vi "Untitled 1 (SubVI).vi"(0 "Message Maker in":refnum<class "Message Maker.lvclass">) -> (19 "error out":errorcluster)   [LabVIEW 2023]
uses:
  Message Maker.lvclass
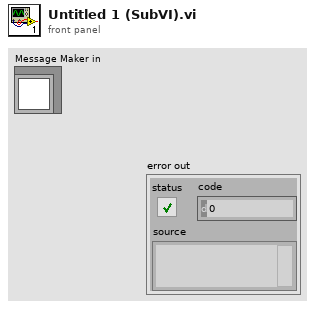
[diagram p1: front panel]
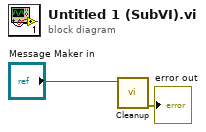
[diagram p0: block diagram]
diagram:
  n1 = call "Cleanup.vi"("Message Maker in"="Message Maker in") -> ("error out"=→"error out":errorcluster)  [unwired: 10 in]
